vi "Bellows Offset Test.vi"() -> ()   [LabVIEW 2020]
uses:
  Classes/Workspace/Workspace.ctl
  Classes/Workspace/Pick Up Tool Area/Pick Up Tool Fixture.lvclass
  Classes/Controller/Controller.lvclass
  Classes/Routine/Pick and Place/Pick and Place.lvclass
  Classes/Controller/Motion/Motion.lvclass
  Classes/Workspace/Fixture.lvclass
panel:
  out "Bellows Center":dbl[](array[numeric])
  out "Workspace Out":T1
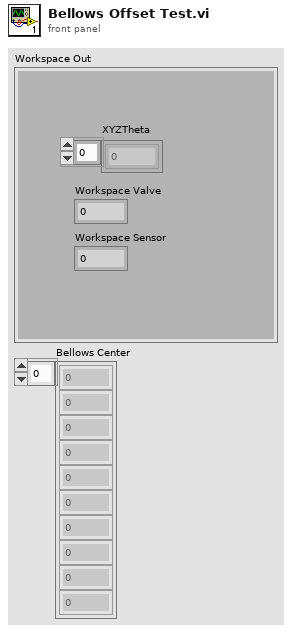
[diagram p1: front panel]
types:
  T1 = typedef "Fixture.lvclass/Workspace.ctl" = cluster{"XYZTheta":dbl[], "Workspace Valve":i32, "Workspace Sensor":i32}
  T2 = typedef "Controller.lvclass/Controllers.ctl" = cluster{"I-O.lvclass":refnum<class "I-O.lvclass">, "Dispenser.lvclass":refnum<class "Dispenser.lvclass">, "Gantry":refnum<k24>}
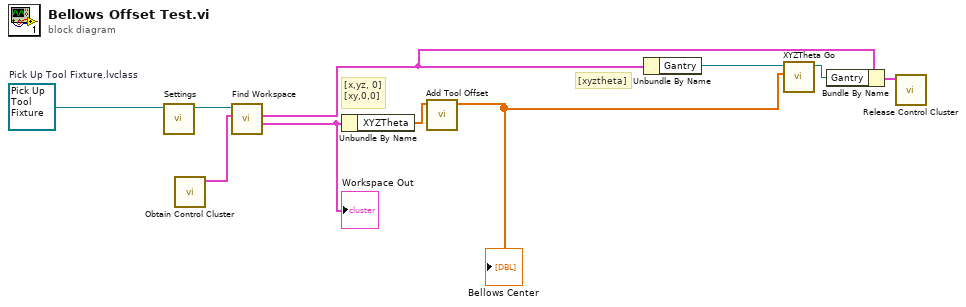
[diagram p0: block diagram]
diagram:
  w10 = refnum<class "Pick Up Tool Fixture.lvclass"> refnum  # Pick Up Tool Fixture.lvclass
  # "[xyztheta]"
  # "[x,yz, 0]\n[xy,0,0]"
  n1 = call-dynamic "Settings.vi"("Workspace in"=w10) -> ("Workspace out"=w9:refnum<class "Pick Up Tool Fixture.lvclass">)  [unwired: 9 in, 1 out]
  n2 = call "Obtain Control Cluster.vi"() -> ("Control Out"=w8:T2)  [unwired: 11 in]
  n3 = call-dynamic "Find Workspace.vi"("Control In"=w8, "Workspace In"=w9) -> ("Workspace Out"=w7:T1, "Control Out"=w5:T2)  [unwired: 6 in, 2 out]
  "Workspace Out" <- w7
  n4 = Unbundle By Name(w7) -> ("XYZTheta"=w6:dbl[])
  n5 = call "Add Tool Offset.vi"("XYZTheta"=w6) -> ("Array"=w1:dbl[])  [unwired: 10 in]
  "Bellows Center" <- w1
  n6 = Unbundle By Name(w5) -> ("Gantry"=w4:refnum<k24>)
  n7 = call "XYZTheta Go.vi"("XYZTheta In"=w1, "Gantry 2"=w4) -> ("Gantry 3"=w3:refnum<k24>)  [unwired: 7 in, 2 out]
  n8 = Bundle By Name(cluster=w5, "Gantry"=w3) -> (w2:T2)
  n9 = call "Release Control Cluster.vi"("output cluster"=w2) -> ()  [unwired: 11 in]
